vi "Arrange VIWin - Arrange BD.vi"(0 "VI in":refnum<vi>, 11 "error in":errorcluster) -> (15 "error out":errorcluster)   [LabVIEW 2020, in "Arrange VI Window.lvlib"]
uses:
  Arrange VI Window.lvlib
  Arrange VIWin - Window Type.ctl
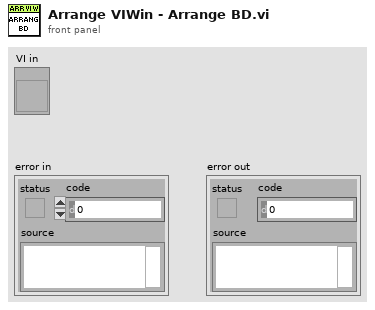
[diagram p1: front panel]
types:
  T1 = typedef "Arrange VI Window.lvlib/Arrange VIWin - Window Type.ctl" = enum16{"FP", "BD"}
  T2 = typedef "LVRectTypeDef.ctl" = cluster{"Left":i16, "Top":i16, "Right":i16, "Bottom":i16}
  T3 = typedef "Arrange VI Window.lvlib/Arrange VIWin - Min Window Dimensions.ctl" = cluster{"min window width":i16, "min window height":i16}
  T4 = typedef "Arrange VI Window.lvlib/Arrange VIWin - Window Gaps.ctl" = cluster{"left gap":i16, "top gap":i16, "min right gap":i16, "min bottom gap":i16}
  T5 = cluster{"display workspace bounds":T2, "min window dimensions":T3, "window gaps":T4}
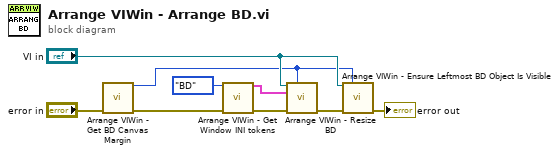
[diagram p0: block diagram]
diagram:
  n1 = call "Arrange VIWin - Get BD Canvas Margin.vi"("error in"="error in") -> ("BD canvas margin"=w4:i16, "error out"=w5:errorcluster)  [unwired: 13 in]
  n2 = call "Arrange VIWin - Get Window INI tokens.vi"("window type"=Arrange_VIWin_-_Window_Type."BD", "error in"=w5) -> ("Window INI tokens"=w1:T5, "error out"=w3:errorcluster)  [unwired: 12 in]
  n3 = call "Arrange VIWin - Resize BD.vi"("VI in"="VI in", "BD canvas margin"=w4, "Window INI tokens"=w1, "error in"=w3) -> ("error out"=w8:errorcluster)  [unwired: 11 in]
  n4 = call "Arrange VIWin - Ensure Leftmost BD Object Is Visible.vi"("VI in"="VI in", "BD canvas margin"=w4, "error in"=w8) -> ("error out"=→"error out":errorcluster)  [unwired: 12 in]
